vi "Draw Dinero FP.vi"(10 "This VI Dinero":refnum<vi>, 11 "Sub Panel Dinero":refnum<vi>) -> ()   [LabVIEW 2020, in "Dinero.lvlib"]
uses:
  Dinero.lvlib
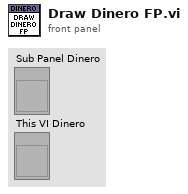
[diagram p1: front panel]
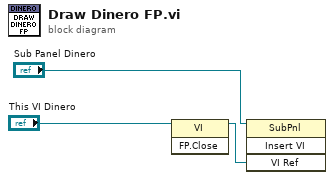
[diagram p0: block diagram]
diagram:
  n1 = invoke class="VI" method="FP.Close"(reference="This VI Dinero") -> (reference out=w3:refnum<vi>)  [unwired: 2 in, 2 out]
  n2 = invoke class="SubPnl" method="Insert VI"(reference="Sub Panel Dinero", "VI Ref"=w3) -> ()  [unwired: 2 in, 4 out]
